vi "ESC UART Read Manual.vi"() -> ()   [LabVIEW 2022 SP3]
doc: "This example performs writes and reads on a serial port, as directed by the user. You can press the Write and Read buttons, and change the Read Count, while the example is running.\n\nThe parameters set for the serial port must match the parameters of the connected instrument or device. In this example, the Read Count parameter specifies the number of bytes that the serial port reads. If there were more bytes at the port than the specified number, those bytes would not be read. If there were less bytes at the port than the specified number, you would receive a timeout error.\n\nThis example expands upon the flow control options for XON and XOFF, allowing the user to choose those control characters. Also, the user can enable or disable a termination character. Some devices require a termination character in order to identify the end of command strings. Some devices send a termination character to signify the end of data to be read. This example shows how you can end the Read operation once a termination character is detected in the buffer and/or append a termination character at the end of the Write data."
uses:
  Program Files/National Instruments/LabVIEW 2022/examples/Instrument IO/Serial/support/Serial - Settings.ctl
  <vilib>/Instr/_visa.llb/VISA Configure Serial Port (Instr).vi
panel:
  out "Status Flag":dbl
  out "Offset":i32
  out "unsigned byte array":u8[](array[numeric])
  out "No Of Errors":i32
  out "N Count":i32
  out "Milliseconds":u32
  out "Happy":bool
  out "Status":bool
  out "error out":errorcluster
  out "Motor Duty Cycle":dbl
  out "Throttle Duty Cycle":dbl
  out "RPM":dbl
  out "Bus Current":dbl
  out "Voltage":dbl
  out "ESC Temperature":dbl
  in  "Read Count/ No. of Bytes":u32=22
  in  "Stop":bool
  in  "Serial Settings":T1={"baud rate"=115200, "data bits"=8, "parity"=enum."None", "stop bits"=10, "flow control"=0} {"flow control" items=["None"=0, "XON/XOFF"=1, "RTS/CTS"=2, "DTR/DSR"=4]; "stop bits" items=["1.0"=10, "1.5"=15, "2.0"=20]; "data bits" min=5 max=8 step=1; "baud rate" items=["75"=75, "110"=110, "134"=134, "150"=150, "300"=300, "600"=600, "1200"=1200, "1800"=1800, "2400"=2400, "4800"=4800, "7200"=7200, "9600"=9600, "14400"=14400, "19200"=19200, "28800"=28800, "38400"=38400, "56000"=56000, "57600"=57600, "115200"=115200, "128000"=128000, "230400"=230400]}
  in  "VISA resource name":refnum<visa-resource-name>="COM19"
  # "Overview: Reads ESC Data from UART Pins + FTDI Cable (Converts UART to Serial). \nAPD HV PRO 240a:\nNumber of Bytes = 22\nBaudrate 115200\nData Bits = 8\nParity = None\nStop Bits = 1.0\nFlow Control = None"
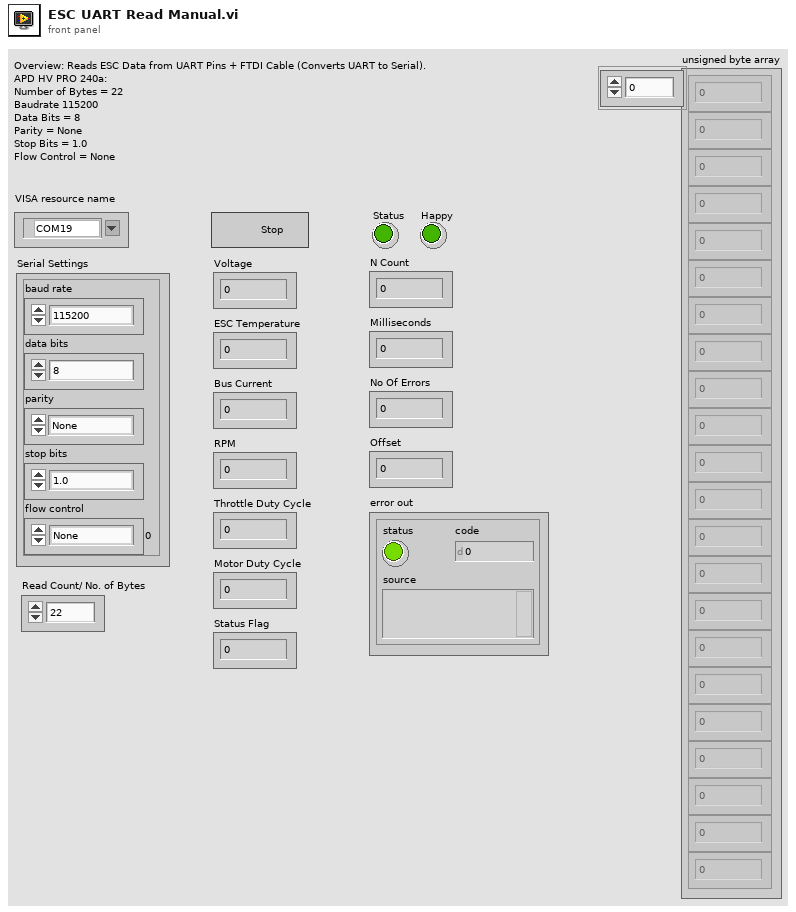
[diagram p1: front panel]
types:
  T1 = typedef "Serial - Settings.ctl" = cluster{"baud rate":u32, "data bits":u16, "parity":enum16{"None", "Odd", "Even", "Mark", "Space"}, "stop bits":u16, "flow control":u16}
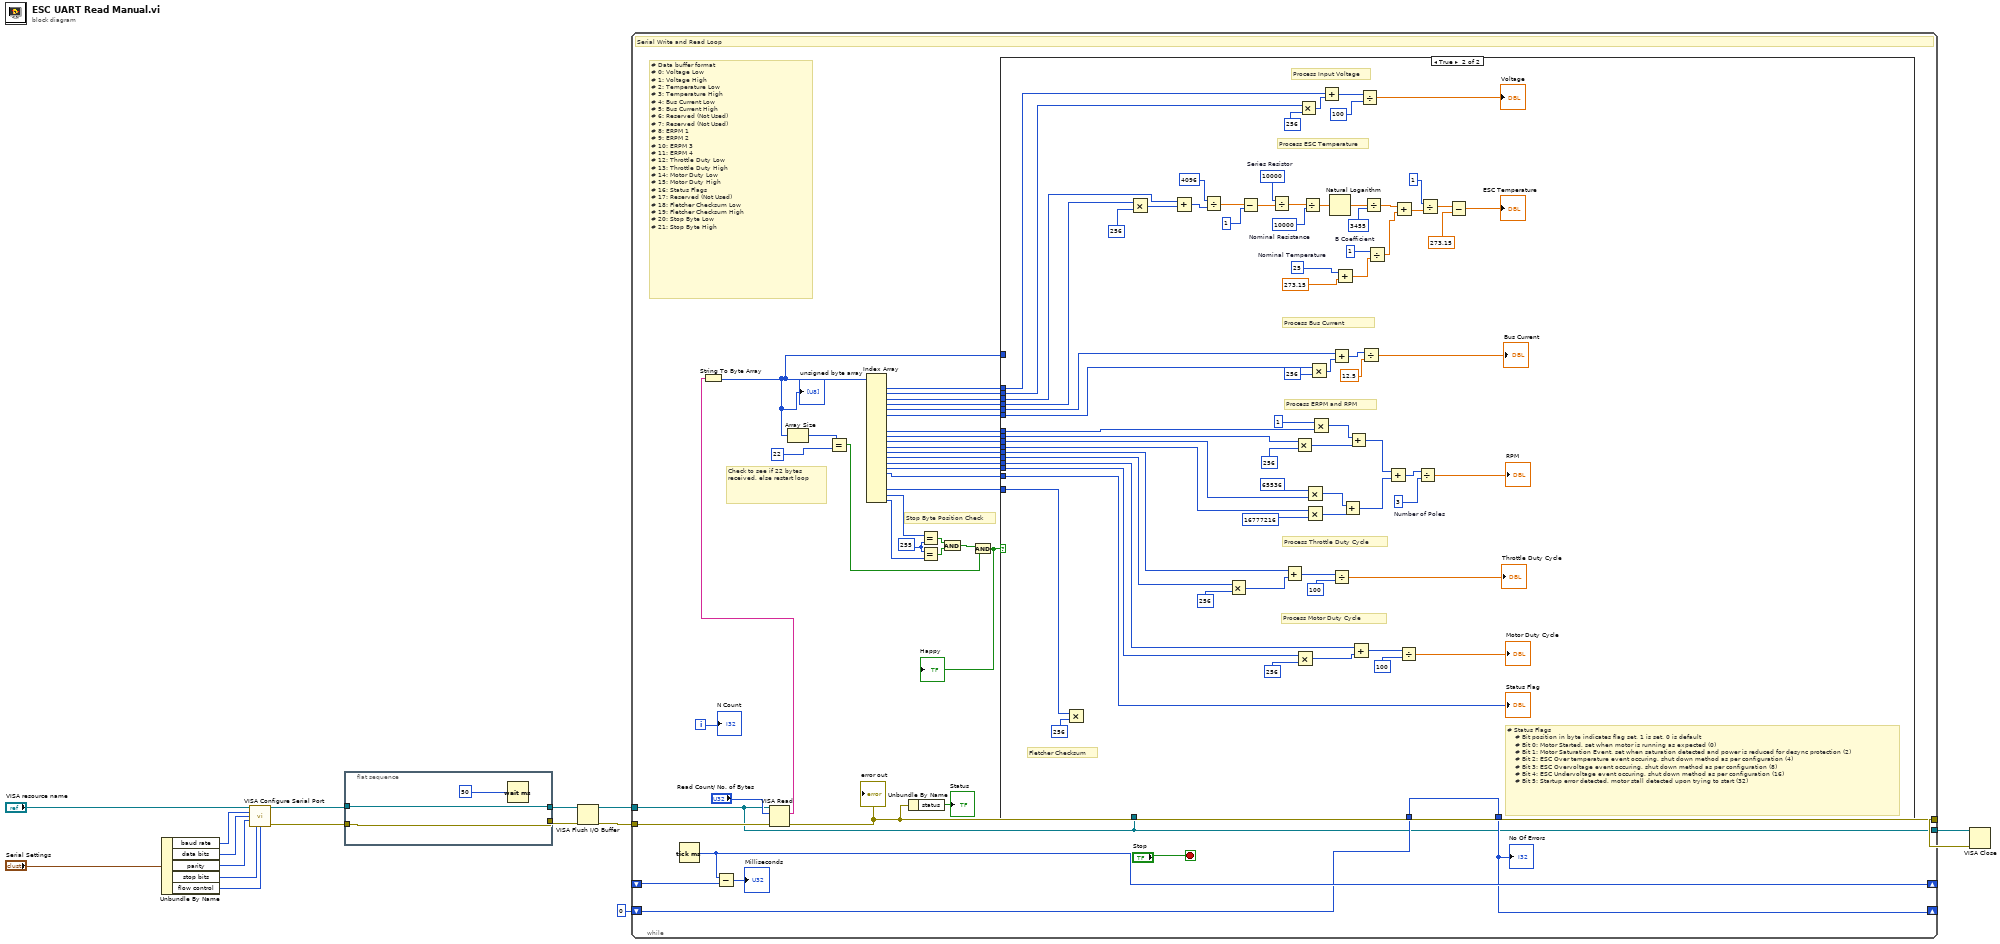
[diagram p0: block diagram]
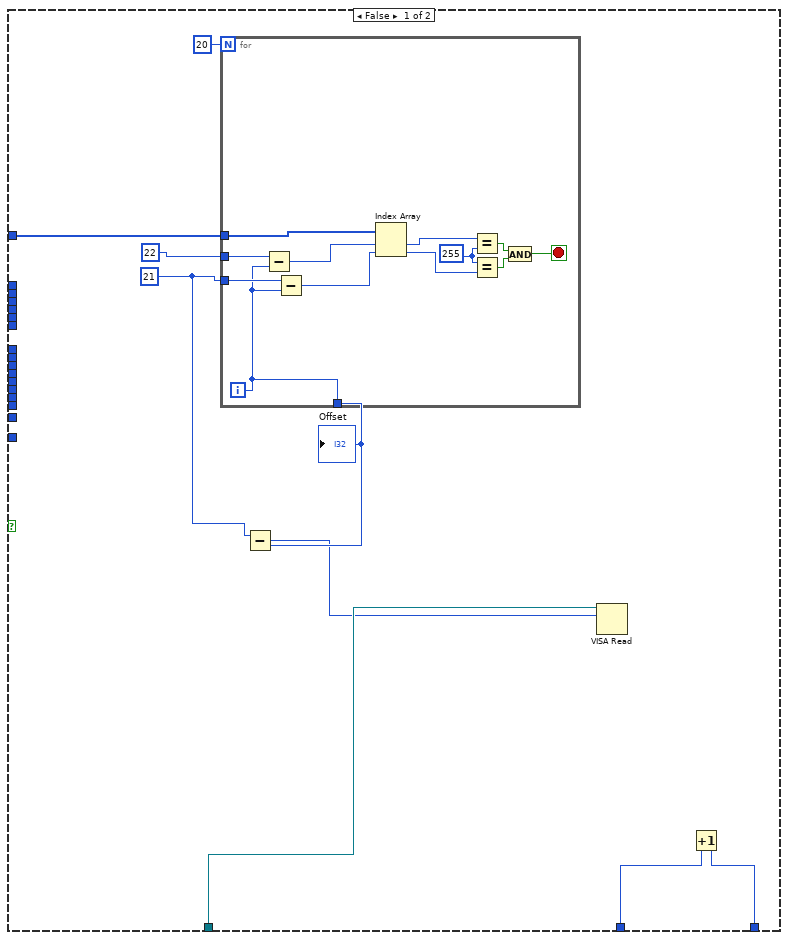
[diagram p2: hidden frame]
diagram:
  n1 = Unbundle By Name("Serial Settings") -> ("baud rate"=w12:u32, "data bits"=w13:u16, "parity"=w14:enum16{"None", "Odd", "Even", "Mark", "Space"}, "stop bits"=w15:u16, "flow control"=w10:u16)
  n2 = call-poly "VISA Configure Serial Port"("VISA resource name"="VISA resource name", "baud rate (9600)"=w12, "data bits (8)"=w13, "parity (0:none)"=w14, "stop bits (10: 1 bit)"=w15, "flow control (0:none)"=w10) -> ("VISA resource name out"=w9:refnum<visa-resource-name>, "error out"=w8:errorcluster)  [unwired: 4 in, 4 out]
  n3 = flat-sequence {
    tunnel: w9 -> [w18]
    tunnel: [w18] -> w7
    tunnel: w8 -> [w17]
    tunnel: [w17] -> w4
    frame #0 {
      n4 = Wait (ms)(milliseconds to wait=50) -> ()  [unwired: 1 out]
    }
  }
  n5 = VISA Flush I/O Buffer(VISA resource name=w7, error in (no error)=w4) -> (VISA resource name out=w6:refnum<visa-resource-name>, error out=w5:errorcluster)  [unwired: 1 in]
  n6 = while {
    tunnel: w5 -> [w51]
    tunnel: w6 -> [w21]
    tunnel: [w21] -> w3
    tunnel: [w30] -> w2
    shift-right: [w27] -> _
    shift-left: _ -> [w28]
    shift-right: [w23] -> _
    shift-left: 0 -> [w24]
    i -> [w25]
    stop <- "Stop" stop-if-true
    w54 = u8 255 ("y")
    # "Stop Byte Position Check"
    # "Check to see if 22 bytes received, else restart loop"
    # "# Data buffer format\n# 0: Voltage Low \n# 1: Voltage High\n# 2: Temperature Low \n# 3: Temperature High\n# 4: Bus Current Low\n# 5: Bus Current High\n# 6: Reserved (Not Used)\n# 7: Reserved (Not Used)\n# 8: ERPM 1\n# 9: ERPM 2\n# 10: ERPM 3\n# 11: ERPM 4\n# 12: Throttle Duty Low\n# 13: Throttle Duty High\n# 14: Motor Duty Low\n# 15: Motor Duty High\n# 16: Status Flags\n# 17: Reserved (Not Used)\n# 18: Fletcher Checksum Low\n# 19: Fletcher Checksum High\n# 20: Stop Byte Low\n# 21: Stop Byte High"
    # "Serial Write and Read Loop"
    n7 = Tick Count (ms)() -> (millisecond timer value=w27:u32)
    n8 = Subtract(x=w27, y=w28) -> (x-y=→"Milliseconds":u32)
    n9 = VISA Read(VISA resource name=w21, byte count="Read Count/ No. of Bytes", error in (no error)=w51) -> (read buffer=w37:string, error out=w30:errorcluster)  [unwired: 2 out]
    "error out" <- w30
    n10 = String To Byte Array(string=w37) -> (unsigned byte array=w22:u8[])
    "unsigned byte array" <- w22
    n11 = Array Size(array=w22) -> (size(s)=w35:i32)
    n12 = Equal?(x=w35, y=22) -> (x = y?=w33:bool)
    n13 = Index Array(array=w22) -> (element #1=w48:u8, element #2=w49:u8, element #3=w58:u8, element #4=w59:u8, element #5=w46:u8, element #6=w47:u8, element #9=w42:u8, element #10=w45:u8, element #11=w44:u8, element #12=w43:u8, element #13=w41:u8, element #14=w40:u8, element #15=w39:u8, element #16=w38:u8, element #17=w20:u8, element #20=w50:u8, element #21=w53:u8, element #22=w55:u8)  [unwired: 22 in, 4 out]
    n14 = Unbundle By Name(w30) -> ("status"=→"Status":bool)
    n15 = Equal?(x=w53, y=w54) -> (x = y?=w56:bool)
    n16 = Equal?(x=w54, y=w55) -> (x = y?=w57:bool)
    n17 = And(x=w56, y=w57) -> (x .and. y?=w34:bool)
    n18 = And(x=w34, y=w33) -> (x .and. y?=w32:bool)
    "Happy" <- w32
    n19 = case shown="True" w32 {
      tunnel: w59 -> [_ w155]
      tunnel: w58 -> [_ w154]
      tunnel: w50 -> [_ w128]
      tunnel: w49 -> [_ w126]
      tunnel: w48 -> [_ w125]
      tunnel: w47 -> [_ w116]
      tunnel: w46 -> [_ w115]
      tunnel: w45 -> [_ w111]
      tunnel: w44 -> [_ w104]
      tunnel: w43 -> [_ w103]
      tunnel: w42 -> [_ w102]
      tunnel: w41 -> [_ w95]
      tunnel: w40 -> [_ w94]
      tunnel: w39 -> [_ w84]
      tunnel: w38 -> [_ w83]
      tunnel: w24 -> [w68 w82]
      tunnel: [w67 w82] -> w23
      tunnel: w22 -> [w66 _]
      tunnel: w21 -> [w63 _]
      tunnel: w20 -> [_ w81]
      frame False {
        w62 = 21 ("index")
        n20 = for {
          N: 20 -> [_]
          tunnel: w66 -> [w80]
          tunnel: 22 ("index") -> [w79]
          tunnel: w62 -> [w77]
          tunnel: [w69] -> w61
          i -> [w69]
          stop <- w70 stop-if-true
          w73 = u8 255 ("y")
          n21 = Subtract(x=w79, y=w69) -> (x-y=w78:i32)
          n22 = Subtract(x=w77, y=w69) -> (x-y=w76:i32)
          n23 = Index Array(array=w80, index #1=w78, index #2=w76) -> (element #1=w72:u8, element #2=w71:u8)
          n24 = Equal?(x=w72, y=w73) -> (x = y?=w74:bool)
          n25 = Equal?(x=w73, y=w71) -> (x = y?=w75:bool)
          n26 = And(x=w74, y=w75) -> (x .and. y?=w70:bool)
        }
        "Offset" <- w61
        n27 = Subtract(x=w62, y=w61) -> (x-y=w60:i32)
        n28 = VISA Read(VISA resource name=w63, byte count=w60) -> ()  [unwired: 1 in, 4 out]
        n29 = Increment(x=w68) -> (x+1=w67:i32)
      }
      frame True {
        w98 = 3  # Number of Poles
        w141 = 25  # Nominal Temperature
        w145 = 3455  # B Coefficient
        w146 = 10000  # Nominal Resistance
        w149 = 10000  # Series Resistor
        # "# Status Flags\n    # Bit position in byte indicates flag set, 1 is set, 0 is default\n    # Bit 0: Motor Started, set when motor is running as expected (0)\n    # Bit 1: Motor Saturation Event, set when saturation detected and power is reduced for desync protection (2)\n    # Bit 2: ESC Over temperature event occuring, shut down method as per configuration (4)\n    # Bit 3: ESC Overvoltage event occuring, shut down method as per configuration (8)\n    # Bit 4: ESC Undervoltage event occuring, shut down method as per configuration (16)\n    # Bit 5: Startup error detected, motor stall detected upon trying to start (32)"
        # "Fletcher Checksum"
        # "Process Motor Duty Cycle"
        # "Process Throttle Duty Cycle"
        # "Process ERPM and RPM"
        # "Process Bus Current"
        # "Process Input Voltage"
        # "Process ESC Temperature"
        n30 = Multiply(x=w128, y=256) -> ()  [unwired: 1 out]
        n31 = Multiply(x=w155, y=256) -> (x*y=w130:i32)
        n32 = Add(x=w154, y=w130) -> (x+y=w153:i32)
        n33 = Divide(x=4096, y=w153) -> (x/y=w151:dbl)
        n34 = Multiply(x=w94, y=256) -> (x*y=w93:i32)
        n35 = Subtract(x=w151, y=1) -> (x-y=w148:dbl)
        n36 = Divide(x=w149, y=w148) -> (x/y=w147:dbl)
        n37 = Add(x=w95, y=w93) -> (x+y=w92:i32)
        n38 = Multiply(x=w111, y=256) -> (x*y=w109:i32)
        n39 = Multiply(x=w83, y=256) -> (x*y=w88:i32)
        n40 = Multiply(x=w126, y=256) -> (x*y=w124:i32)
        n41 = Divide(x=w147, y=w146) -> (x/y=w133:dbl)
        n42 = Multiply(x=65536 ("y"), y=w104) -> (x*y=w106:i32)
        n43 = Multiply(x=w103, y=16777216) -> (x*y=w105:i32)
        n44 = Multiply(x=w116, y=256) -> (x*y=w120:i32)
        n45 = Multiply(x=1 ("y"), y=w102) -> (x*y=w110:i32)
        n46 = Add(x=w125, y=w124) -> (x+y=w123:i32)
        n47 = Natural Logarithm(1:w133) -> (0:w132:dbl)
        n48 = Add(x=w115, y=w120) -> (x+y=w119:i32)
        n49 = Divide(x=w92, y=100) -> (x/y=→"Throttle Duty Cycle":dbl)
        n50 = Add(x=w141, y=273.15) -> (x+y=w140:dbl)
        n51 = Add(x=w106, y=w105) -> (x+y=w101:i32)
        n52 = Add(x=w110, y=w109) -> (x+y=w100:i32)
        n53 = Add(x=w84, y=w88) -> (x+y=w87:i32)
        n54 = Divide(x=w123, y=100) -> (x/y=→"Voltage":dbl)
        n55 = Divide(x=w119, y=12.5) -> (x/y=→"Bus Current":dbl)
        n56 = Divide(x=w132, y=w145) -> (x/y=w144:dbl)
        n57 = Divide(x=1, y=w140) -> (x/y=w139:dbl)
        n58 = Add(x=w100, y=w101) -> (x+y=w99:i32)
        n59 = Add(x=w144, y=w139) -> (x+y=w138:dbl)
        n60 = Divide(x=w87, y=100) -> (x/y=→"Motor Duty Cycle":dbl)
        n61 = Divide(x=w99, y=w98) -> (x/y=→"RPM":dbl)
        n62 = Divide(x=1, y=w138) -> (x/y=w136:dbl)
        n63 = Subtract(x=w136, y=273.15) -> (x-y=→"ESC Temperature":dbl)
        "Status Flag" <- w81
      }
    }
    "No Of Errors" <- w23
    "N Count" <- w25
  }
  n64 = VISA Close(VISA resource name=w3, error in (no error)=w2) -> ()  [unwired: 1 out]
